vi "EventBuilder.read DAQ data.vi"(0 "i ref in":refnum<vi>, 2 "eventID":i32, 3 "ms timeout (10000)":i32=10000, 5 "error in (no error)":errorcluster) -> (14 "i ref out":refnum<vi>, 17 "timed out":bool, 19 "error out":errorcluster)   [LabVIEW 2014, in "EventBuilder.lvlib"]
doc: "reads the data from the specified DAQ objects and puts it into the internal buffer of THIS class."
uses:
  EventBuilder.lvlib
  CS_Core/CSSystem/CoreDefs/CoreDefs.error_type.ctl
  CS_Core/CSSystem/CoreDefs/CoreDefs.rawDataType.ctl
  CS_Core/CSSystem/CoreDefs/CoreDefs.error_severity.ctl
  CS_Core/BaseProcess/BaseProcess.descriptor string definition.ctl
  CS_Core/CSSystem/CoreLib/CoreLib.lvlib
  CS_Core/BaseProcess/BaseProcess.lvlib
  DataLib/DataLib.lvlib
  CS_Core/CSSystem/CSSystemLib/CSSystemLib.lvlib
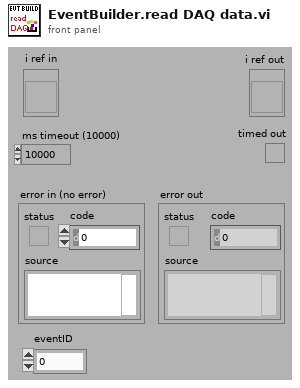
[diagram p1: front panel]
types:
  T1 = typedef "CoreDefs.error_type.ctl" = enum16{"no error", "can't load process", "can't unload process", "process does not exist", "can't install process", "can't remove process", "unknown function", "time out", "can't execute function", "duplicate queue name", "super not found", "caller queue invalid", "can't ping process", "unknown error", "VISA Error", "VISA timeout", "GPIB timeout", "GPIB error", "communication error", "data type mismatch", "can't read data from OPC server", "can't write data to OPC server", "OET error", "function not implemented", "process already exists", "invalid Shared Variable name", "error writing Shared Variable", "error reading Shared Variable", "invalid client name", "corrupt database", "unknown class", "call not authorized", "parameter out of range", "OET timeout: can't get data to modify", "invalid queue name", "requested operation incompatible with current state", "event undefined", "event disabled", "state undefined", "caller is not a friend", "EventBuilder: bad eventID", "EventBuilder: no DAQ devices", "a thread must not stop itself", "UNUSED ELEMENT4", "DiscArchiver: eventData incomplete", "DiscArchiver: eventData does not belong to run", "DiscArchiver: can't open file", "DiscArchiver: can't write to file", "DiscArchiver: available disc space low", "can't acquire semaphore", "error reading data from database", "notifier object is not existing", "can't register process", "can't unregister process", "illegal event type", "object disabled", "object already exists", "can't change state", "Instrument not found", "no connection to remote node", "invalid reference", "N/A", "UNUSED ELEMENT 1", "element not found", "illegal TCP/IP connection detected", "object does not exist", "invalid access ID", "unknown CS system", "invalid privilige", "unsupported data type", "unsupported server type", "IO server already exists", "Shared Variable already exists"}
  T2 = typedef "CoreDefs.rawDataType.ctl" = i8[]
  T3 = typedef "CoreDefs.error_severity.ctl" = enum16{"undefined", "information", "warning", "error", "fatal"}
  T4 = typedef "BaseProcess.lvlib/BaseProcess.descriptor string definition.ctl" = string
  T5 = typedef "EventBuilder.lvlib/EventBuilder.i attribute.ctl" = cluster{"header":string, "DAQObjs":string[], "headerID":dbl, "eventID":i32, "dataDescriptionID":i32, "eventDataID":i32, "eventDataSize":i32, "dataDescriptionSize":i32}
  T6 = typedef "CoreDefs.call_type.ctl" = cluster{"Object":string, "Selector":string, "CallType":enum16{"simple", "synchronous", "asynchronous"}, "Async Object":string, "Async Selector":string, "Data Descriptor":T4, "Data":T2, "Error #":i32, "Expire":u32}
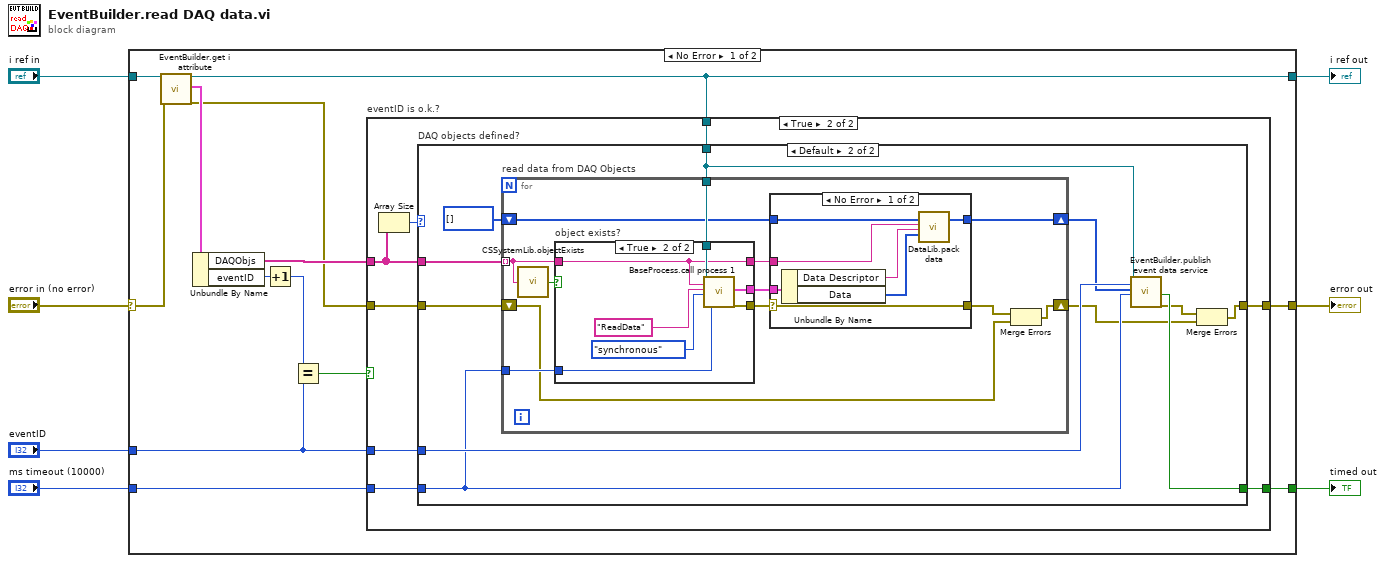
[diagram p0: block diagram]
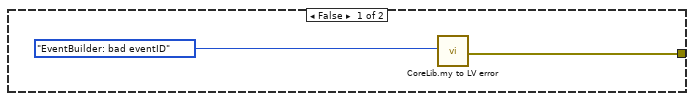
[diagram p2: hidden frame]
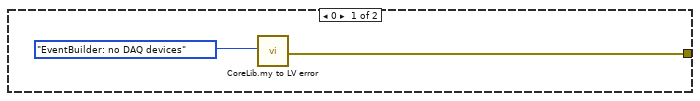
[diagram p3: hidden frame]
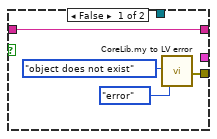
[diagram p4: hidden frame]
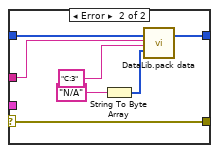
[diagram p5: hidden frame]
diagram:
  n1 = case shown="No Error" "error in (no error)" {
    selector: "error in (no error)" -> [w18 w81]
    tunnel: "i ref in" -> [w20 w82]
    tunnel: "ms timeout (10000)" -> [w10 _]
    tunnel: "eventID" -> [w12 _]
    tunnel: [w8 w81] -> w4
    tunnel: [w15 w82] -> w3
    tunnel: [w9 _] -> w1
    frame No Error {
      n2 = call "EventBuilder.get i attribute.vi"("i ref in"=w20, "error in (no error)"=w18) -> ("i ref out"=w15:refnum<vi>, "i attribute"=w19:T5, "error out"=w16:errorcluster)  [unwired: 15 in]
      n3 = Unbundle By Name(w19) -> ("DAQObjs"=w17:string[], "eventID"=w14:i32)
      n4 = Increment(x=w14) -> (x+1=w13:i32)
      n5 = Equal?(x=w13, y=w12) -> (x = y?=w11:bool)
      n6 = case "eventID is o.k.?" shown="True" w11 {
        tunnel: [w21 w30] -> w8
        tunnel: w17 -> [_ w29]
        tunnel: w15 -> [_ w28]
        tunnel: w16 -> [_ w27]
        tunnel: w12 -> [_ w26]
        tunnel: w10 -> [_ w24]
        tunnel: [_ w23] -> w9
        frame False {
          n7 = call "CoreLib.my to LV error.vi"("ErrorTypes"=CoreDefs.error_type."EventBuilder: bad eventID") -> ("myErrorCluster"=w21:errorcluster)  [unwired: 17 in, 1 out]
        }
        frame True {
          n8 = Array Size(array=w29) -> (size(s)=w25:i32)
          n9 = case "DAQ objects defined?" shown="Default" w25 {
            tunnel: [w31 w33] -> w30
            tunnel: w29 -> [_ w42]
            tunnel: w28 -> [_ w40]
            tunnel: w27 -> [_ w43]
            tunnel: w26 -> [_ w39]
            tunnel: w24 -> [_ w36]
            tunnel: [_ w37] -> w23
            frame 0 {
              n10 = call "CoreLib.my to LV error.vi"("ErrorTypes"=CoreDefs.error_type."EventBuilder: no DAQ devices") -> ("myErrorCluster"=w31:errorcluster)  [unwired: 17 in, 1 out]
            }
            frame Default {
              n11 = for "read data from DAQ Objects" {
                tunnel: w42 -> [w47] mode=indexing
                tunnel: w40 -> [w55]
                shift-right: [w44] -> w35
                shift-left: w43 -> [w45]
                shift-right: [w53] -> w38
                shift-left: T2 [] ("Array") -> [w54]
                tunnel: w36 -> [w52]
                n12 = call "CSSystemLib.objectExists.vi"("name"=w47) -> ("obj exists"=w48:bool)
                n13 = case "object exists?" shown="True" w48 {
                  tunnel: w55 -> [_ w66]
                  tunnel: w47 -> [w59 w60]
                  tunnel: w52 -> [_ w65]
                  tunnel: [_ w64] -> w51
                  tunnel: [w58 w61] -> w50
                  tunnel: [w59 w60] -> w49
                  frame False {
                    n14 = call "CoreLib.my to LV error.vi"("ErrorTypes"=CoreDefs.error_type."object does not exist", "severityLevel"=CoreDefs.error_severity."error") -> ("myErrorCluster"=w58:errorcluster)  [unwired: 16 in, 1 out]
                  }
                  frame True {
                    n15 = call "BaseProcess.call process 1.vi"("i ref in"=w66, "Object"=w60, "Selector"="ReadData", "CallType"=enum16{"simple", "synchronous", "asynchronous"}."synchronous", "timeout (ms)"=w65) -> ("call cluster out"=w64:T6, "error out"=w61:errorcluster)  [unwired: 12 in, 1 out]
                  }
                }
                n16 = case shown="No Error" w50 {
                  selector: w50 -> [w72 w80]
                  tunnel: w51 -> [w73 _]
                  tunnel: [w72 w80] -> w46
                  tunnel: w49 -> [w70 w76]
                  tunnel: w54 -> [w71 w78]
                  tunnel: [w67 w77] -> w53
                  frame No Error {
                    n17 = Unbundle By Name(w73) -> ("Data Descriptor"=w69:T4, "Data"=w68:T2)
                    n18 = call "DataLib.pack data.vi"("dataIn"=w71, "DAQDevice"=w70, "Data Descriptor"=w69, "DAQDeviceData"=w68) -> ("dataOut"=w67:T2)  [unwired: 15 in]
                  }
                  frame Error {
                    n19 = String To Byte Array(string="N/A") -> (unsigned byte array=w74:u8[])
                    n20 = call "DataLib.pack data.vi"("dataIn"=w78, "DAQDevice"=w76, "Data Descriptor"=T4 "C:3", "DAQDeviceData"=w74) -> ("dataOut"=w77:T2)  [unwired: 15 in]
                  }
                }
                n21 = Merge Errors(w46, w45) -> (w44:errorcluster)
              }
              n22 = call "EventBuilder.publish event data service.vi"("i ref in"=w40, "eventID"=w39, "eventData"=w38, "ms timeout (10000)"=w36) -> ("timed out"=w37:bool, "error out"=w34:errorcluster)  [unwired: 13 in, 1 out]
              n23 = Merge Errors(w34, w35) -> (w33:errorcluster)
            }
          }
        }
      }
    }
    frame Error {
    }
  }
  "error out" <- w4
  "i ref out" <- w3
  "timed out" <- w1
